vi "3_3_Face_Detection_Inference(FPGA)(Cam).vi"() -> ()   [LabVIEW 2020]
doc: "This example demonstrates the usage of the \"DeepLTK FPGA Addon\" for deploying a Face Detection model on a PXI-FPGA board, utilizing an input image sourced from a camera. \n\nMore Examples: https://github.com/ngenehub/deepltk_fpga_examples"
uses:
  <vilib>/Ngene/DeepLTK FPGA Addon/Toolkit/NNF_Host/Low_Level/NNF_Init/Controls/NNF_FPGA_Target_Info.ctl
  <vilib>/userDefined/High Color/nirio_resource_hc.ctl
  <vilib>/vision/driver/IMAQdx.llb/IMAQdx Camera Control Mode.ctl
  <vilib>/vision/driver/IMAQdx.llb/IMAQdx Buffer Number Mode.ctl
  <vilib>/Ngene/DeepLTK FPGA Addon/Toolkit/NNF_Host/API/NNF_Set_Input/NNF_Set_Input(2D_U32).vi
  <vilib>/Ngene/DeepLTK FPGA Addon/Toolkit/NNF_Host/Low_Level/NNF_Set_Input/NNF_Copy_Data_to_Buffer(U64).vi
  <vilib>/Ngene/DeepLTK FPGA Addon/Toolkit/NNF_Host/Low_Level/NNF_Set_Input/NNF_Copy_Data_to_Buffer(U32).vi
  <vilib>/FPGAPlugInAG/Dynamic/niLvFpga_Download_Dynamic.vi
  <vilib>/FPGAPlugInAG/Dynamic/niLvFpga_Run_Dynamic.vi
  <vilib>/Ngene/DeepLTK FPGA Addon/Toolkit/NNF_Host/Low_Level/NNF_Forward/NNF_Get_CPU_Subnet_Data_from_Variant.vi
  <vilib>/Ngene/Deep Learning Toolkit/Toolkit/NN_Network/API/NN_Set_Input.vi
  <vilib>/Ngene/Deep Learning Toolkit/Toolkit/NN_Network/API/NN_Set_Input/3D/NN_Set_Input(3D_SGL_idx).vi
  <vilib>/Ngene/DeepLTK FPGA Addon/Toolkit/NNF_Host/Low_Level/NNF_Common/SubVIs/NNF_GLobal.vi
  <vilib>/FPGAPlugInAG/Dynamic/niLvFpga_Close_Dynamic.vi
  <vilib>/rvi/interface/nirviMethod/nirviMethod.xnode
  <vilib>/rvi/interface/nirviCloseFPGA/nirviCloseFPGA.xnode
  <vilib>/vision/driver/NI_Vision_Acquisition_Software.lvlib
  <resource>/objmgr/imaqdx.rc
  <vilib>/vision/NI_Vision_Development_Module.lvlib
  <vilib>/Ngene/DeepLTK FPGA Addon/Toolkit/DeepLTK_FPGA_Addon.lvlib
  <vilib>/Ngene/Deep Learning Toolkit/Toolkit/Deep_Learning_Toolkit_by_Ngene.lvlib
  <vilib>/ptbypt/NI_PtbyPt.lvlib
panel:
  in  "FPGA Bitfile":path=path "D:/Ngene/GitHub/deepltk_fpga_examples/FPGA Bitfiles/NNF_sbRIO_9609_8Cores.lvbitx"
  in  "FPGA Target":T1="rio://10.0.0.39/RIO0" caption="RIO Device"
  out "Target Information":T2={"BRAM _Buff_1_Size"=52500, "BRAM _Buff_2_Size"=45937, "Version"=[8, 1, 1, 0], "# Cores"=8}
  out "Loop time":dbl=0.03711719999955676 format="%#_4p"
  out "Inference time":dbl=0.028291524999931424 format="%#_4p"
  out "Display":T3(plugin-control)
  in  "Confidence_Thresh":sgl=0.39999998
  in  "IOU_Thresh":sgl=0.3
  in  "Camera":refnum<k21>="cam0" caption="IMAQdx Session"
  in  "Weight File Path":path=path "D:/Ngene/GitHub/deepltk_fpga_examples/2_Face_Detection(PXI,sbRIO)/Models/Face_Detection_NNF_Converted/NNF_Face_Detection.bin"
  in  "Configuration File Path":path=path "D:/Ngene/GitHub/deepltk_fpga_examples/2_Face_Detection(PXI,sbRIO)/Models/Face_Detection_NNF_Converted/NNF_Face_Detection.cfg"
  in  "Scalers File Path":path=path "D:/Ngene/GitHub/deepltk_fpga_examples/2_Face_Detection(PXI,sbRIO)/Models/Face_Detection_NNF_Converted/NNF_Face_Detection_Scalers.cfg"
  in  "Stop":bool
  in  "Camera Resolution":i32(listbox)
  # "Overview: \nThis example demonstrates the usage of the \"DeepLTK FPGA Addon\" for deploying a Face Detection model on a PXI-FPGA board, utilizing an input image sourced from a camera.\nRequirements: \n• DeepLTK - Deep Learning Toolkit for LabVIEW (https://www.ngene.co/deep-learning-toolkit-for-labview)\n• DeepLTK FPGA Addon (https://www.ngene.co/deepltk-accelerator-for-fpga)\n• Vision Development Module\n• NI FPGA Module\n• Web Camera"
  # "Instructions:\nNote: To run the example on RT target copy converted model  and FPGA bitfile to the RT target. \n1.\tSelect FPGA target at FPGA Target control.\n2.\tProvide path to compiled FPGA bitfile at FPGA Bitfile control. A sample is available in the \"Examples\\FPGA Bitfiles\" folder. \n3. Provide paths to .cfg, .bin and scalers.cfg files generated during model conversion or sample from project (locted in \"Models\\Face_Detection_NNF_Converted\" folder ) at Network Configuration File Path, Weight File Path and Scalers File Path controls.. \n4. Select the camera from \"Camera\" control.\n5. Run the VI. \n6. Observe the detections drawn on the \"Display\". The info on the top left of each bounding box represents detected object class and the confidence level.\nMore Examples: https://github.com/ngenehub/deepltk_fpga_examples"
  # "Copy resource path from NI MAX if needed"
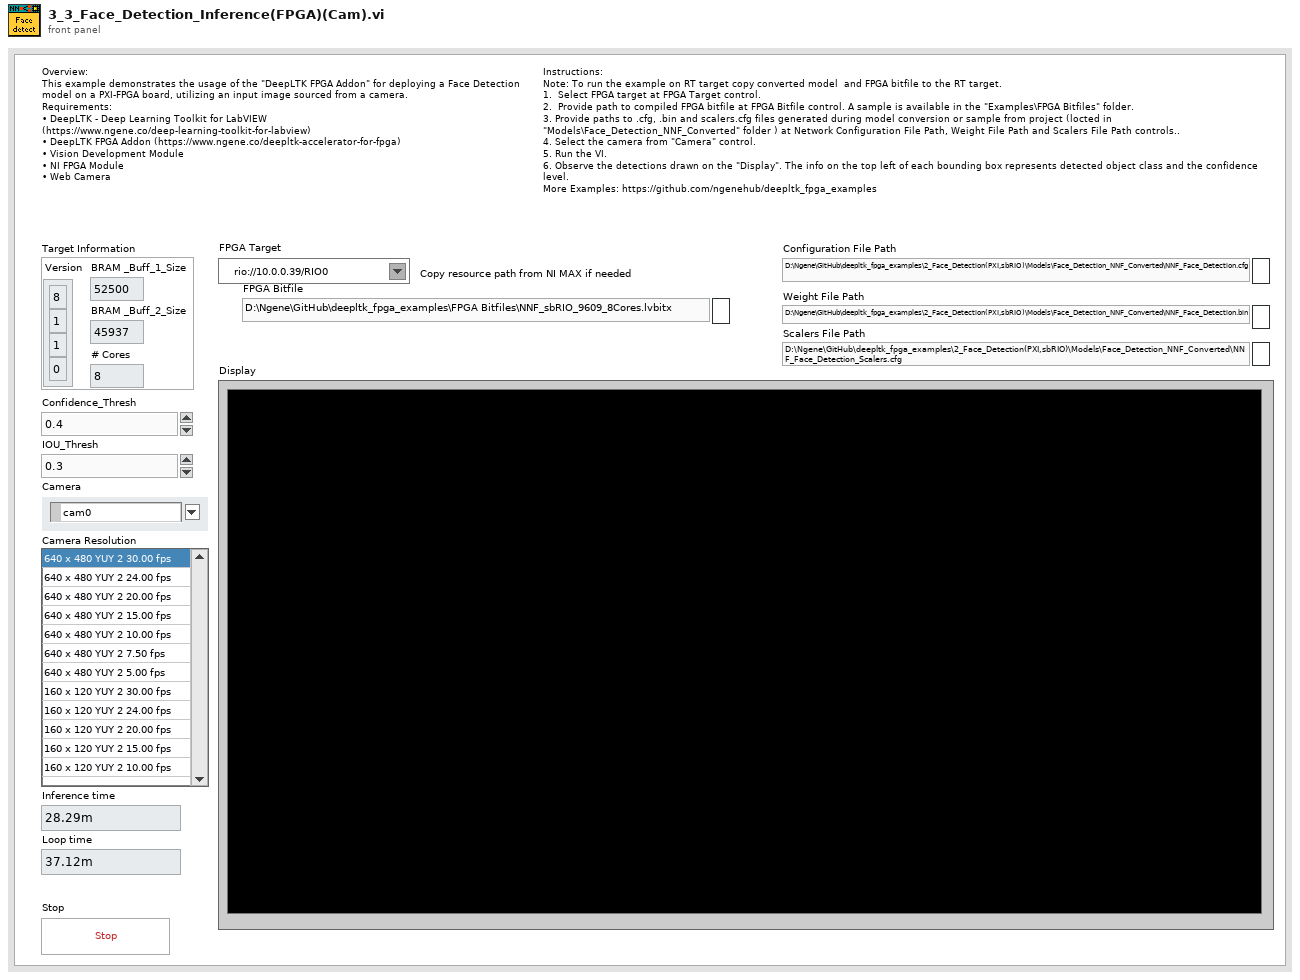
[diagram p1: front panel]
types:
  T1 = typedef "nirio_resource_hc.ctl" = tag
  T2 = typedef "DeepLTK_FPGA_Addon.lvlib/NNF_FPGA_Target_Info.ctl" = cluster{"BRAM _Buff_1_Size":u32, "BRAM _Buff_2_Size":u32, "Version":u8[], "# Cores":u32}
  T3 = typedef "IMAQ Image.ctl" = refnum<image>
  T4 = typedef "Image Type" = u32
  T5 = typedef "NI_Vision_Acquisition_Software.lvlib/IMAQdx Camera Control Mode.ctl" = enum32{"Controller", "Listener"}
  T6 = typedef "IMAQdx.ctl" = refnum<k21>
  T7 = typedef "DeepLTK_FPGA_Addon.lvlib/NNF.ctl" = cluster{"FPGA VI Ref ":refnum<k20>, "Subnets":T8[], "Dims_In":T10, "#Cores(enum)":T11, "NN_Ref":T12}
  T8 = typedef "DeepLTK_FPGA_Addon.lvlib/NNF_Subnet.ctl" = cluster{"Subnet Type":T9, "Subnet Data":variant, "Input Scaler":sgl, "Output Scaler":sgl}
  T9 = typedef "DeepLTK_FPGA_Addon.lvlib/NNF_Subnet_Type.ctl" = enum16{"CPU", "FPGA", "Split FPGA"}
  T10 = typedef "Deep_Learning_Toolkit_by_Ngene.lvlib/NN_Dims(C,H,W).ctl" = cluster{"C":i32, "H":i32, "W":i32}
  T11 = typedef "DeepLTK_FPGA_Addon.lvlib/NNF_No_Of_Cores.ctl" = enum16{"4CH", "8CH"}
  T12 = typedef "DeepLTK_FPGA_Addon.lvlib/NN_DVR.ctl" = refnum<data-value>
  T13 = typedef "Deep_Learning_Toolkit_by_Ngene.lvlib/NN.ctl" = cluster{"Name":string, "No of Layers":i32, "mBatch":i32, "Layers":T14[], "Dimty":T15, "Dims_In":T10, "Dims_Out":T10, "Working_Dir":path, "Train?":bool, "Train_Params":T16, "LR_Update_Policy":T19, "Session Data":T21, "Ground_truth":T22, "NNg_hdls":T23, "NN_Device":T24, "GPU Id":i32, "Labels":string[], "Receptive Field":T25[], "Loss_Type":T26, "Loss_Cfg_Prms":variant, "NNG_WS":T27}
  T14 = typedef "Deep_Learning_Toolkit_by_Ngene.lvlib/NN_Layer_ref.ctl" = refnum<data-value>
  T15 = typedef "Deep_Learning_Toolkit_by_Ngene.lvlib/NN_In_Out_Dim-ty.ctl" = enum8{"In1D_Out1D", "In3D_Out1D", "In3D_Out3D", "In3D_OutBBox"}
  T16 = typedef "Deep_Learning_Toolkit_by_Ngene.lvlib/NN_Train_Params.ctl" = cluster{"Optimizer":T17, "Beta_1":sgl, "Beta_2":sgl, "Weight Decay(L1)":sgl, "Weight Decay(L2)":sgl, "Data_Sampling":T18}
  T17 = typedef "Deep_Learning_Toolkit_by_Ngene.lvlib/NN_Train_Optimizer.ctl" = enum16{"SGD", "Adam", "Adagrad", "Adadelta", "RMSProp", "Nesterov"}
  T18 = typedef "Deep_Learning_Toolkit_by_Ngene.lvlib/NN_Train_Data_Sampling.ctl" = enum16{"Random", "Sequential"}
  T19 = typedef "Deep_Learning_Toolkit_by_Ngene.lvlib/NN_LR_Policy_Cfg.ctl" = cluster{"Policy_Type":T20, "LR0":dbl, "k":sgl, "WarmUp_Policy":enum16{"Step", "Ramp"}, "WarmUp_Iter":i32, "WarmUp_Ratio":sgl}
  T20 = typedef "Deep_Learning_Toolkit_by_Ngene.lvlib/NN_LR_Policy_Type.ctl" = enum16{"Manual", "Step", "Exp", "1/t"}
  T21 = typedef "Deep_Learning_Toolkit_by_Ngene.lvlib/NN_Train_Session_Data.ctl" = cluster{"Epochs":sgl, "Tot_Iter":i32, "LR":sgl, "LR_iter":i32}
  T22 = typedef "Deep_Learning_Toolkit_by_Ngene.lvlib/NN_Ground_truth.ctl" = cluster{"Y":variant}
  T23 = typedef "Deep_Learning_Toolkit_by_Ngene.lvlib/nng_cuda_handles.ctl" = cluster{"cudnn":u64, "cublas":u64, "stream":u64, "curand":u64}
  T24 = typedef "Deep_Learning_Toolkit_by_Ngene.lvlib/NN_Device.ctl" = enum16{"CPU", "GPU"}
  T25 = typedef "Deep_Learning_Toolkit_by_Ngene.lvlib/NN_Dims(V,H).ctl" = cluster{"V":i32, "H":i32}
  T26 = typedef "Deep_Learning_Toolkit_by_Ngene.lvlib/NN_Loss_Type.ctl" = enum16{"None", "MSE", "CrossEntropy", "YOLO_v2", "YOLO_v4"}
  T27 = typedef "Deep_Learning_Toolkit_by_Ngene.lvlib/NNG_WS.ctl" = cluster{"NNG_WS_Mem":T28, "Max_WS_Size":i64}
  T28 = typedef "Deep_Learning_Toolkit_by_Ngene.lvlib/NNg_WS_Mem_DVR.ctl" = refnum<data-value>
  T29 = typedef "NI_Vision_Acquisition_Software.lvlib/IMAQdx Buffer Number Mode.ctl" = enum32{"Next", "Last", "Buffer Number", "Every", "Last New"}
  T30 = typedef "Deep_Learning_Toolkit_by_Ngene.lvlib/NN_Layer.ctl" = cluster{"Name":string, "Layer_Data":variant, "Layer_Type":T31, "Dims_In":T10, "Layers_In":variant, "Dims_Out":T10, "Layers_Out":variant, "Metrics":T32, "GPU_Data":variant, "mBatch":i32, "NN_Device":T24, "NNg_hdls":T23, "Train?":bool, "Dimty":T33, "RecptField":T34}
  T31 = typedef "Deep_Learning_Toolkit_by_Ngene.lvlib/NN_Layer_Type.ctl" = enum16{"Input1D", "Input3D", "Conv1D", "Conv2D", "Conv2D_Adv", "MaxPool", "AvgPool", "UpSample", "DropOut3D", "ShortCut", "Concat", "SoftMax3D", "FC", "DropOut", "Softmax", "Flatten", "YOLO_v2", "YOLO_v4", "Activation", "BatchNormalization", "Unsupported"}
  T32 = typedef "Deep_Learning_Toolkit_by_Ngene.lvlib/NN_Layer_Metrics.ctl" = cluster{"Data":dbl, "Params":dbl, "Ops":dbl}
  T33 = typedef "Deep_Learning_Toolkit_by_Ngene.lvlib/NN_Layer_Dimty.ctl" = enum16{"1D", "3D"}
  T34 = typedef "Deep_Learning_Toolkit_by_Ngene.lvlib/NN_Layer_RF_State.ctl" = cluster{"Dims":T25, "J":T25}
  T35 = typedef "Deep_Learning_Toolkit_by_Ngene.lvlib/NN_BBox_Detection.ctl" = cluster{"Class":i32, "Conf Level":sgl, "BBox":T36}
  T36 = typedef "Deep_Learning_Toolkit_by_Ngene.lvlib/NN_BBox.ctl" = cluster{"x":sgl, "y":sgl, "w":sgl, "h":sgl}
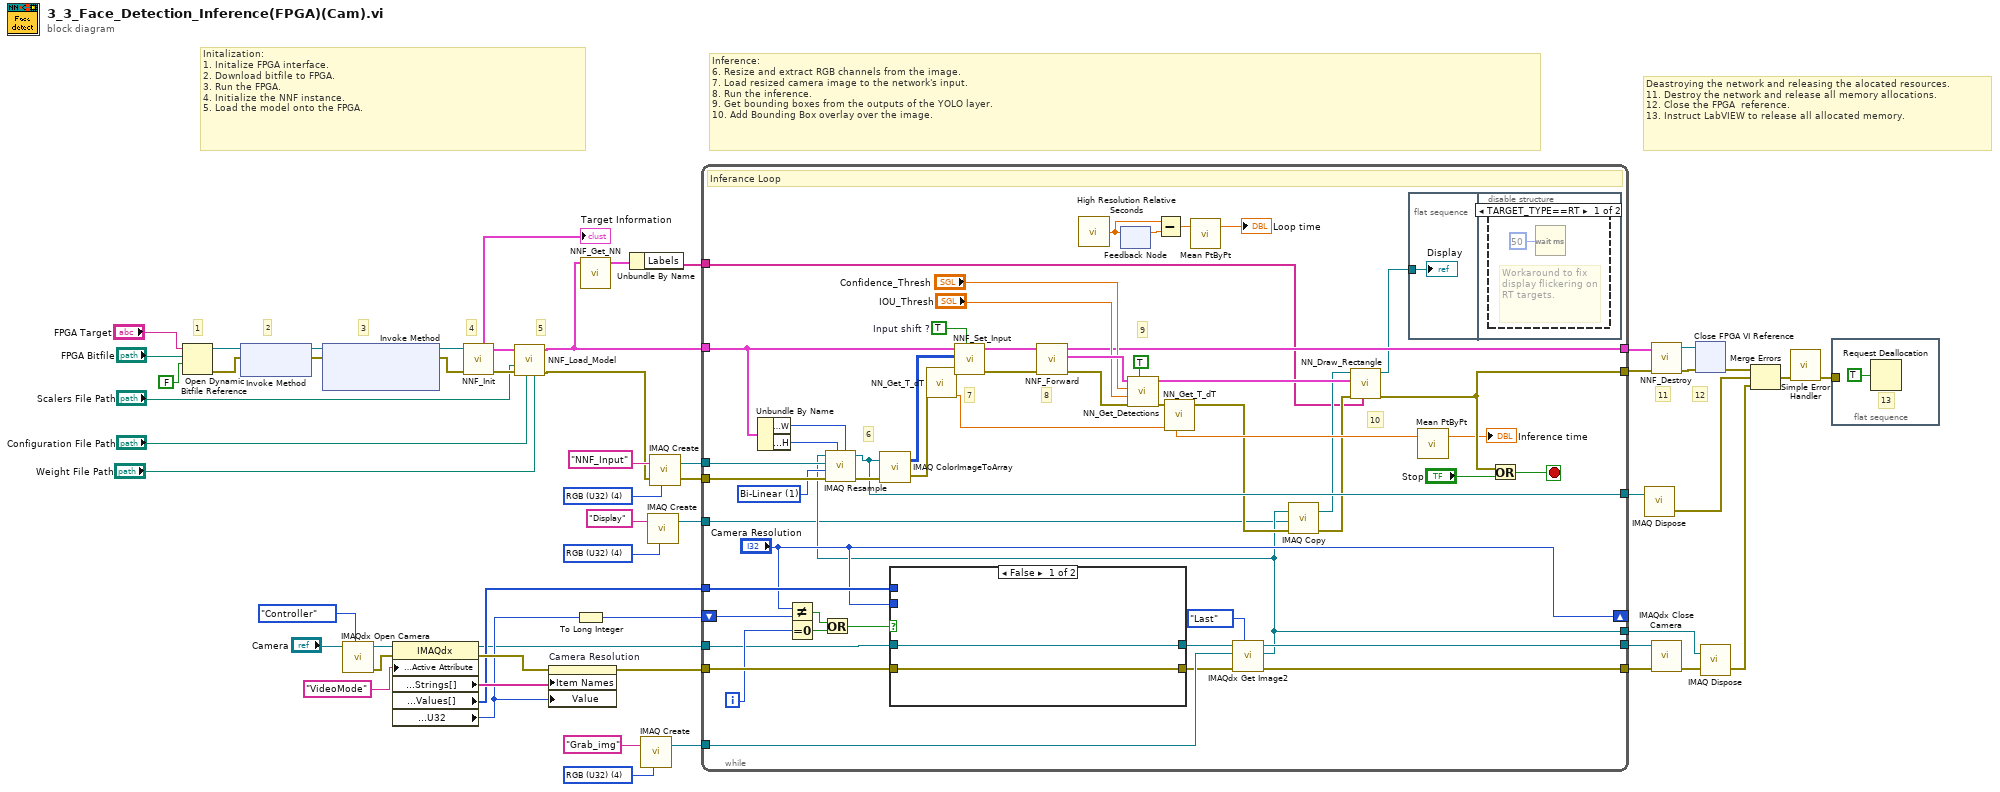
[diagram p0: block diagram]
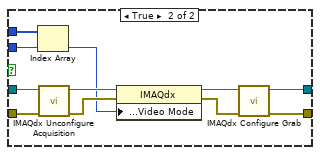
[diagram p3: hidden frame]
diagram:
  w4 = T4 4 items=["Grayscale (U8)", "Grayscale (I16)", "Grayscale (SGL)", "Complex (CSG)", "RGB (U32)", "HSL (U32)", "RGB (U64)", "Grayscale (U16)"] ("Image Type")
  w7 = T4 4 items=["Grayscale (U8)", "Grayscale (I16)", "Grayscale (SGL)", "Complex (CSG)", "RGB (U32)", "HSL (U32)", "RGB (U64)", "Grayscale (U16)"] ("Image Type")
  w40 = T4 4 items=["Grayscale (U8)", "Grayscale (I16)", "Grayscale (SGL)", "Complex (CSG)", "RGB (U32)", "HSL (U32)", "RGB (U64)", "Grayscale (U16)"] ("Image Type")
  # "12"
  # "11"
  # "Deastroying the network and releasing the alocated resources. \n11. Destroy the network and release all memory allocations.\n12. Close the FPGA  reference.\n13. Instruct LabVIEW to release all allocated memory."
  # "Inference:\n6.\tResize and extract RGB channels from the image.\n7.\tLoad resized camera image to the network's input.\n8.\tRun the inference.\n9.\tGet bounding boxes from the outputs of the YOLO layer. \n10. Add Bounding Box overlay over the image."
  # "5"
  # "4"
  # "3"
  # "2"
  # "1"
  # "Initalization:\n1. Initalize FPGA interface.\n2. Download bitfile to FPGA.\n3. Run the FPGA.\n4. Initialize the NNF instance.\n5. Load the model onto the FPGA."
  n1 = Open Dynamic Bitfile Reference(0:"FPGA Target", 1:"FPGA Bitfile", 2:FALSE ("Run When Loaded")) -> (5:w22:refnum<k20>, 8:w18:errorcluster)  [unwired: 2 in]
  n2 = xnode "Invoke Method"("FPGA VI Reference In"=w22, "error in"=w18) -> ("FPGA VI Reference Out"=w19:refnum<k20>, "error out"=w16:errorcluster)
  n3 = xnode "Invoke Method"("FPGA VI Reference In"=w19, "error in"=w16) -> ("FPGA VI Reference Out"=w17:refnum<k20>, "error out"=w15:errorcluster)  [unwired: 1 in]
  n4 = call <vilib>:"IMAQdx Open Camera.vi"("Camera Control Mode"=IMAQdx_Camera_Control_Mode."Controller", "Session In"="Camera") -> ("error out"=w49:errorcluster, "Session Out"=w51:T6)  [unwired: 1 in, 7 out]
  n5 = property class="IMAQdx"(reference=w51, error in=w49, "Camera Attributes:Active Attribute"="VideoMode" ("ActiveAttribute")) -> (reference out=w42:T6, error out=w48:errorcluster, "Camera Attributes:Enum:Strings[]"=w47:string[], "Camera Attributes:Enum:Values[]"=w44:u32[], "Camera Attributes:Value:U32"=w46:u32)
  n6 = call <vilib>:"NNF_Init.vi"("error in"=w15, "FPGA Interface"=w17) -> ("error out"=w23:errorcluster, "NNF out"=w21:T7, "Target Information"=→"Target Information":T2)  [unwired: 7 in]
  n7 = call <vilib>:"NNF_Load_Model.vi"("Weight File Path"="Weight File Path", "Network CFG File Path"="Configuration File Path", "Error in"=w23, "Scalers"="Scalers File Path", "NNF in"=w21) -> ("error Out"=w14:errorcluster, "NNF out"=w1:T7)  [unwired: 5 in]
  n8 = property on="Camera Resolution" class="LstBox (strict)"(error in=w48, "Item Names"=w47, "Value"=w46) -> (error out=w41:errorcluster)  [unwired: 1 in, 1 out]
  n9 = To Long Integer(number=w46) -> (32bit integer=w43:i32)
  n10 = call "NNF_Get_NN.vi"("NNF in"=w1) -> ("NN out"=w3:T13)  [unwired: 10 in]
  n11 = Unbundle By Name(w3) -> ("Labels"=w2:string[])
  n12 = call "IMAQ Create"("Image Name"="Grab_img", "Image Type"=w4) -> ("New Image"=w55:T3)  [unwired: 3 in, 1 out]
  n13 = call "IMAQ Create"("Image Name"="Display", "Image Type"=w7) -> ("New Image"=w5:T3)  [unwired: 3 in, 1 out]
  n14 = call "IMAQ Create"("Image Name"="NNF_Input", "Image Type"=w40, "error in (no error)"=w14) -> ("New Image"=w52:T3, "error out"=w38:errorcluster)  [unwired: 2 in]
  n15 = while {
    tunnel: w1 -> [w71]
    tunnel: w44 -> [w107]
    tunnel: w55 -> [w97]
    tunnel: w52 -> [w102]
    tunnel: [w58] -> w37
    tunnel: [w77] -> w36
    shift-right: ["Camera Resolution"] -> _
    shift-left: w43 -> [w105]
    tunnel: w42 -> [w98]
    tunnel: w41 -> [w106]
    tunnel: w38 -> [w103]
    tunnel: [w64] -> w33
    tunnel: [w76] -> w32
    tunnel: [w61] -> w30
    tunnel: [w75] -> w29
    tunnel: w5 -> [w60]
    tunnel: w2 -> [w57]
    i -> [w104]
    stop <- w109 stop-if-true
    w70 = TRUE  # Input shift ?
    w86 = u32 1 items=["Zero Order", "Bi-Linear", "Quadratic", "Cubic Spline"] ("Interpolation Type")
    # "7"
    # "6"
    # "10"
    # "9"
    # "8"
    # "Inferance Loop"
    n16 = Unbundle By Name(w71) -> ("Dims_In.W"=w87:i32, "Dims_In.H"=w88:i32)
    n17 = Not Equal?(x="Camera Resolution", y=w105) -> (x != y?=w93:bool)
    n18 = Equal To 0?(x=w104) -> (x = 0?=w92:bool)
    n19 = Or(x=w93, y=w92) -> (x .or. y?=w94:bool)
    n20 = case shown="False" w94 {
      tunnel: w98 -> [w113 w122]
      tunnel: w106 -> [w112 w121]
      tunnel: [w113 w118] -> w91
      tunnel: [w112 w119] -> w90
      tunnel: w107 -> [_ w124]
      tunnel: "Camera Resolution" -> [_ w123]
      frame False {
      }
      frame True {
        n21 = Index Array(array=w124, index=w123) -> (element=w114:u32)
        n22 = call <vilib>:"IMAQdx Unconfigure Acquisition.vi"("error in"=w121, "Session In"=w122) -> ("error out"=w115:errorcluster, "Session Out"=w120:T6)  [unwired: 8 out]
        n23 = property class="IMAQdx"(reference=w120, error in=w115, "Acquisition Attributes:Video Mode"=w114) -> (reference out=w117:T6, error out=w116:errorcluster)
        n24 = call <vilib>:"IMAQdx Configure Grab.vi"("error in"=w116, "Session In"=w117) -> ("error out"=w119:errorcluster, "Session Out"=w118:T6)  [unwired: 2 in, 6 out]
      }
    }
    n25 = call <vilib>:"High Resolution Relative Seconds.vi"() -> ("relative seconds"=w74:dbl)
    n26 = feedback #1() -> (w73:dbl)  [unwired: 1 in]
    n27 = feedback-in #1(w74) -> ()
    n28 = Subtract(x=w74, y=w73) -> (x-y=w72:dbl)
    n29 = call <vilib>:"Mean PtByPt.vi"("x"=w72) -> ("mean"=→"Loop time":dbl)  [unwired: 3 in, 1 out]
    n30 = call <vilib>:"IMAQdx Get Image2.vi"("Buffer Number Mode (Next)"=IMAQdx_Buffer_Number_Mode."Last", "error in"=w90, "Image In"=w97, "Session In"=w91) -> ("error out"=w64:errorcluster, "Image Out"=w61:T3, "Session Out"=w76:T6)  [unwired: 4 in, 1 out]
    n31 = call "IMAQ Resample"("X Resolution"=w87, "Y Resolution"=w88, "error in (no error)"=w103, "Interpolation Type"=w86, "Image Dst"=w102, "Image Src"=w61) -> ("error out"=w89:errorcluster, "Image Dst Out"=w75:T3)  [unwired: 4 in]
    n32 = call "IMAQ ColorImageToArray"("Image"=w75, "error in (no error)"=w89) -> ("Image Pixels (U32)"=w96:u32[][], "error out"=w99:errorcluster)  [unwired: 2 in, 1 out]
    n33 = call <vilib>:"NN_Get_T_dT.vi"("error in (no error)"=w99) -> ("T_out"=w68:dbl, "error out"=w69:errorcluster)  [unwired: 6 in, 1 out]
    n34 = call-poly <vilib>:"NNF_Set_Input.vi"("Input shift ?"=w70, "error in"=w69, "Data_in(2D_U32)"=w96, "NNF in"=w71) -> ("error out"=w100:errorcluster, "NNF out"=w101:T7)  [unwired: 6 in]
    n35 = call <vilib>:"NNF_Forward.vi"("error in"=w100, "NNF in"=w101) -> ("error out"=w80:errorcluster, "Last_Layer"=w81:T30, "NNF out"=w58:T7)  [unwired: 7 in]
    n36 = call <vilib>:"NN_Get_Detections.vi"("Temporal Averaging (F)"=TRUE, "error in"=w80, "IOU_Thrsh"="IOU_Thresh", "Confidence_Thrsh"="Confidence_Thresh", "YOLO_Layer"=w81) -> ("error out"=w83:errorcluster, "Detections"=w82:T35[])  [unwired: 5 in]
    n37 = call <vilib>:"NN_Get_T_dT.vi"("T_in"=w68, "error in (no error)"=w83) -> ("error out"=w62:errorcluster, "dT"=w67:dbl)  [unwired: 5 in, 1 out]
    n38 = call "IMAQ Copy"("error in (no error)"=w62, "Image Dst"=w60, "Image Src"=w61) -> ("error out"=w59:errorcluster, "Image Dst Out"=w63:T3)  [unwired: 3 in]
    n39 = call "NN_Draw_Rectangle.vi"("Labels"=w57, "error in (no error)"=w59, "Draw_Boxes"=w82, "Image_in"=w63) -> ("error out"=w77:errorcluster, "Image_out"=w56:T3)  [unwired: 5 in, 1 out]
    n40 = flat-sequence {
      tunnel: w56 -> [w110]
      frame #0 {
        "Display" <- w110
      }
      frame #1 {
        n41 = disable-structure shown="TARGET_TYPE==RT" {
          frame condition #0 {
            # "Workaround to fix display flickering on RT targets."
            n42 = Wait (ms)(milliseconds to wait=u32 50) -> ()  [unwired: 1 out]
          }
          frame condition #1 (active) {
          }
        }
      }
    }
    n43 = call <vilib>:"Mean PtByPt.vi"("x"=w67) -> ("mean"=→"Inference time":dbl)  [unwired: 3 in, 1 out]
    n44 = Or(x=w77, y="Stop") -> (x .or. y?=w109:bool)
  }
  n45 = call "IMAQ Dispose"("Image"=w29) -> ("error out"=w27:errorcluster)  [unwired: 5 in]
  n46 = call <vilib>:"NNF_Destroy.vi"("error in"=w36, "NNF in"=w37) -> ("error out"=w34:errorcluster, "FPGA VI Ref"=w24:refnum<k20>)  [unwired: 8 in]
  n47 = call <vilib>:"IMAQdx Close Camera.vi"("error in"=w33, "Session In"=w32) -> ("error out"=w31:errorcluster)  [unwired: 9 out]
  n48 = xnode "Close FPGA VI Reference"("FPGA VI Reference In"=w24, "error in"=w34) -> ("error out"=w25:errorcluster)
  n49 = call "IMAQ Dispose"("Image"=w30, "error in (no error)"=w31) -> ("error out"=w26:errorcluster)  [unwired: 4 in]
  n50 = Merge Errors(w25, w27, w26) -> (w28:errorcluster)
  n51 = call <vilib>:"Simple Error Handler.vi"("error in (no error)"=w28) -> ("error out"=w39:errorcluster)  [unwired: 4 in, 4 out]
  n52 = flat-sequence {
    tunnel: w39 -> [_]
    frame #0 {
      # "13"
      n53 = Request Deallocation(TRUE ("flag")) -> ()
    }
  }
